vi "reverse imageU16.vi"(0 "output array in":u16[][](array[numeric]), 1 "reverse v":bool, 2 "reverse h":bool) -> (3 "output array out":u16[][](array[numeric]))   [LabVIEW 2024]
uses:
  <vilib>/vision/NI_Vision_Development_Module.lvlib
panel:
  out "x-y":dbl
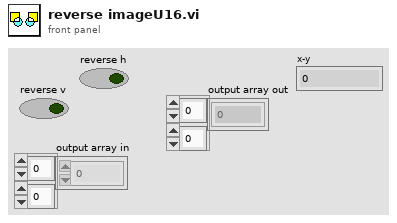
[diagram p1: front panel]
types:
  T1 = typedef "Image Type" = u32
  T2 = typedef "IMAQ Image.ctl" = refnum<image>
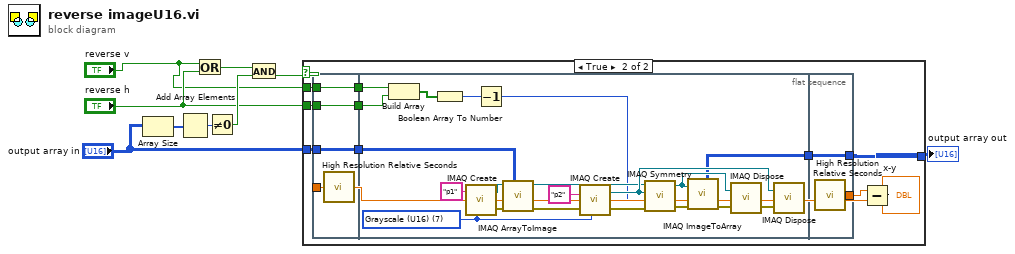
[diagram p0: block diagram]
diagram:
  n1 = Array Size(array="output array in") -> (size(s)=w7:i32[])
  n2 = Add Array Elements(numeric array=w7) -> (sum=w6:i32)
  n3 = Or(x="reverse v", y="reverse h") -> (x .or. y?=w4:bool)
  n4 = Not Equal To 0?(x=w6) -> (x != 0?=w3:bool)
  n5 = And(x=w4, y=w3) -> (x .and. y?=w5:bool)
  n6 = case shown="True" w5 {
    tunnel: [w10 w20] -> w9
    tunnel: "output array in" -> [w10 w21]
    tunnel: "reverse v" -> [_ w19]
    tunnel: "reverse h" -> [_ w18]
    frame False {
    }
    frame True {
      n7 = flat-sequence {
        tunnel: w18 -> [w23]
        tunnel: w19 -> [w24]
        tunnel: w21 -> [w25]
        tunnel: [w25] -> w17
        tunnel: [w24] -> w16
        tunnel: [w23] -> w15
        tunnel: [w22] -> w11
        tunnel: w17 -> [w32]
        tunnel: w16 -> [w30]
        tunnel: w15 -> [w29]
        tunnel: [w31] -> w14
        tunnel: [w47] -> w20
        tunnel: w14 -> [w47]
        tunnel: [w46] -> w13
        frame #0 {
          n8 = call <vilib>:"High Resolution Relative Seconds.vi"() -> ("relative seconds"=w22:dbl)
        }
        frame #1 {
          w34 = T1 7 items=["Grayscale (U8)", "Grayscale (I16)", "Grayscale (SGL)", "Complex (CSG)", "RGB (U32)", "HSL (U32)", "RGB (U64)", "Grayscale (U16)"] ("Image Type")
          n9 = Build Array(w30, w29) -> (w28:bool[])
          n10 = Boolean Array To Number(Boolean array=w28) -> (number=w27:u32)
          n11 = call "IMAQ Create"("Image Name"="p1", "Image Type"=w34) -> ("New Image"=w36:T2, "error out"=w38:errorcluster)  [unwired: 3 in]
          n12 = Decrement(x=w27) -> (x-1=w26:u32)
          n13 = call "IMAQ ArrayToImage"("Image Pixels (U16)"=w32, "error in (no error)"=w38, "Image"=w36) -> ("error out"=w39:errorcluster, "Image Out"=w37:T2)  [unwired: 7 in]
          n14 = call "IMAQ Create"("Image Name"="p2", "Image Type"=w34, "error in (no error)"=w39) -> ("New Image"=w45:T2, "error out"=w40:errorcluster)  [unwired: 2 in]
          n15 = call "IMAQ Symmetry"("error in (no error)"=w40, "Type of Symmetry"=w26, "Image Dst"=w45, "Image Src"=w37) -> ("error out"=w41:errorcluster, "Image Dst Out"=w44:T2)  [unwired: 1 in]
          n16 = call "IMAQ ImageToArray"("error in (no error)"=w41, "Image"=w44) -> ("Image Pixels (U16)"=w31:u16[][], "error out"=w42:errorcluster)  [unwired: 2 in, 3 out]
          n17 = call "IMAQ Dispose"("Image"=w44, "error in (no error)"=w42) -> ("error out"=w43:errorcluster)  [unwired: 4 in]
          n18 = call "IMAQ Dispose"("Image"=w45, "error in (no error)"=w43) -> ()  [unwired: 4 in, 1 out]
        }
        frame #2 {
          n19 = call <vilib>:"High Resolution Relative Seconds.vi"() -> ("relative seconds"=w46:dbl)
        }
      }
      n20 = Subtract(x=w13, y=w11) -> (x-y=→"x-y":dbl)
    }
  }
  "output array out" <- w9
